vi "PPS_TRAJECTORY_EXECUTE_ABS.vi"(8 "Init":bool, 11 "End Pose ENG":T6={"TRANSLATION"={"X"=0.0, "Y"=0.0}, "ROTATION"={"VALUE"=0.0, "COS"=1.0, "SIN"=0.0}} {"ROTATION"."SIN" format="%13.4f"; "ROTATION"."COS" format="%13.4f"; "ROTATION"."VALUE" format="%13.4f"; "TRANSLATION"."Y" format="%14.3f"; "TRANSLATION"."X" format="%14.3f"}) -> (0 "AtReference":bool, 3 "Chassis Velocity Target SI":T7 {"vOmega" format="%10.3f"; "vY" format="%10.3f"; "vX" format="%10.3f"})   [LabVIEW 2019]
uses:
  <vilib>/Rock Robotics/WPI/ThirdParty/JAS_Junk/TrajLib/TypeDef/CHASSIS_SPEEDS.ctl
  <vilib>/Rock Robotics/WPI/ThirdParty/JAS_Junk/TrajLib/TypeDef/POSE2D.ctl
  <vilib>/Rock Robotics/WPI/ThirdParty/JAS_Junk/TrajLib/TypeDef/TRANSLATION2D.ctl
  <vilib>/Rock Robotics/WPI/ThirdParty/JAS_Junk/TrajLib/TypeDef/ROTATION2D.ctl
  <vilib>/Rock Robotics/WPI/ThirdParty/MJansen/PathPlanner/TypeDef/PathPlannerTrajectory.ctl
  <vilib>/Rock Robotics/WPI/ThirdParty/MJansen/PathPlanner/TypeDef/PathPlannerTrajectoryState.ctl
  <vilib>/Rock Robotics/WPI/ThirdParty/MJansen/PathPlanner/TypeDef/PathPlannerPathConstraints.ctl
  <vilib>/Rock Robotics/WPI/ThirdParty/JAS_Junk/TrajLib/VI/Util_GetTime_U32.vi
  <vilib>/Rock Robotics/WPI/ThirdParty/JAS_Junk/TrajLib/ProfiledPIDController_NewPeriod.vi
  <vilib>/Rock Robotics/WPI/ThirdParty/JAS_Junk/TrajLib/ProfiledPIDController_SetIntegratorRange.vi
  <vilib>/Rock Robotics/WPI/ThirdParty/JAS_Junk/TrajLib/ProfiledPIDController_DisableContInput.vi
  <vilib>/Rock Robotics/WPI/ThirdParty/JAS_Junk/TrajLib/ProfiledPIDController_EnableContInput.vi
  <vilib>/Rock Robotics/WPI/ThirdParty/JAS_Junk/TrajLib/TrapProfConstraint_New.vi
  <vilib>/Rock Robotics/WPI/ThirdParty/JAS_Junk/TrajLib/Pose2d_New.vi
  <vilib>/Rock Robotics/WPI/ThirdParty/JAS_Junk/TrajLib/Conv_Deg_Radians.vi
  <vilib>/Rock Robotics/WPI/ThirdParty/JAS_Junk/TrajLib/Rotation2d_UnaryMinus.vi
  <vilib>/Rock Robotics/WPI/ThirdParty/JAS_Junk/TrajLib/Rotation2d_RotateBy.vi
  <vilib>/Rock Robotics/WPI/ThirdParty/JAS_Junk/TrajLib/Rotation2d_GetRadians.vi
  <vilib>/Rock Robotics/WPI/ThirdParty/JAS_Junk/TrajLib/TrapProfState_New.vi
  <vilib>/Rock Robotics/WPI/ThirdParty/JAS_Junk/TrajLib/PIDController_NewPeriod.vi
  <vilib>/Rock Robotics/SystemInterfaces/NetworkCommunication/NetComm_UsageReport_report.vi
  <vilib>/Rock Robotics/WPI/ThirdParty/JAS_Junk/TrajLib/PIDController_SetIntegratorRange.vi
  <vilib>/Rock Robotics/WPI/ThirdParty/JAS_Junk/TrajLib/PIDController_DisableContinousInput.vi
  <vilib>/Rock Robotics/WPI/ThirdParty/JAS_Junk/TrajLib/PIDController_EnableContinousInput.vi
  <vilib>/Rock Robotics/WPI/ThirdParty/JAS_Junk/TrajLib/Rotation2d_CreateAngle.vi
  <vilib>/Rock Robotics/WPI/ThirdParty/JAS_Junk/TrajLib/Translation2d_Create.vi
  <vilib>/Rock Robotics/WPI/ThirdParty/JAS_Junk/TrajLib/Rotation2d_CreateXY.vi
  <vilib>/Rock Robotics/WPI/ThirdParty/JAS_Junk/TrajLib/Util_CalcDist.vi
  <vilib>/Rock Robotics/WPI/ThirdParty/JAS_Junk/TrajLib/VI/Util_GetTime_U64.vi
  PPS_TRAJECTORY_GLOBALS.vi
  Swerve_Drive_System/PPS_DRIVE_GLOBALS.vi
  <vilib>/Rock Robotics/WPI/ThirdParty/JAS_Junk/TrajLib/Globals/Util_LibraryGlobals.vi
  <vilib>/Rock Robotics/WPI/ThirdParty/JAS_Junk/TrajLib/Trajectory_Library.lvlib
  <vilib>/Rock Robotics/WPI/ThirdParty/MJansen/PathPlanner/PathPlanner24.lvlib
panel:
  out "PathPlannerTrajectory":T1 {"States"."TargetHolonomicRotation"."SIN" format="%13.4f"; "States"."TargetHolonomicRotation"."COS" format="%13.4f"; "States"."TargetHolonomicRotation"."VALUE" format="%13.4f"; "States"."Heading"."SIN" format="%13.4f"; "States"."Heading"."COS" format="%13.4f"; "States"."Heading"."VALUE" format="%13.4f"; "States"."PositionMeters"."Y" format="%14.3f"; "States"."PositionMeters"."X" format="%14.3f"}
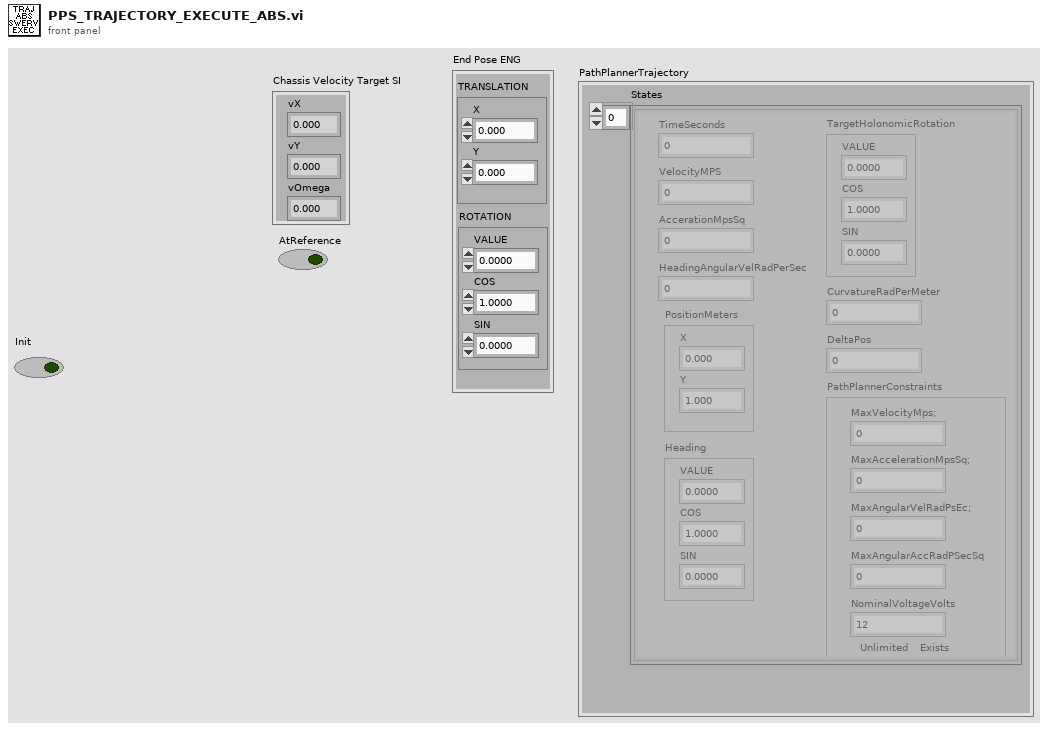
[diagram p1: front panel]
types:
  T1 = typedef "PathPlanner24.lvlib/PathPlannerTrajectory.ctl" = cluster{"States":T2[]}
  T2 = typedef "PathPlanner24.lvlib/PathPlannerTrajectoryState.ctl" = cluster{"TimeSeconds":dbl, "VelocityMPS":dbl, "AccerationMpsSq":dbl, "HeadingAngularVelRadPerSec":dbl, "PositionMeters":T3, "Heading":T4, "TargetHolonomicRotation":T4, "CurvatureRadPerMeter":dbl, "PathPlannerConstraints":T5, "DeltaPos":dbl}
  T3 = typedef "Trajectory_Library.lvlib/TRANSLATION2D.ctl" = cluster{"X":dbl, "Y":dbl}
  T4 = typedef "Trajectory_Library.lvlib/ROTATION2D.ctl" = cluster{"VALUE":dbl, "COS":dbl, "SIN":dbl}
  T5 = typedef "PathPlanner24.lvlib/PathPlannerPathConstraints.ctl" = cluster{"MaxVelocityMps;":dbl, "MaxAccelerationMpsSq;":dbl, "MaxAngularVelRadPsEc;":dbl, "MaxAngularAccRadPSecSq":dbl, "Exists":bool, "Unlimited":bool, "NominalVoltageVolts":dbl}
  T6 = typedef "Trajectory_Library.lvlib/POSE2D.ctl" = cluster{"TRANSLATION":T3, "ROTATION":T4}
  T7 = typedef "Trajectory_Library.lvlib/CHASSIS_SPEEDS.ctl" = cluster{"vX":dbl, "vY":dbl, "vOmega":dbl}
  T8 = typedef "Trajectory_Library.lvlib/SWERVE_DRIVE_KINEMATICS.ctl" = cluster{"NumModules":i32, "InverseKinematics":T9, "ForwardKinematics":T9, "Modules":T3[], "PrevCoR":T3, "SavedModuleStates":T10[]}
  T9 = typedef "NI_Matrix.lvlib/RealMatrix.ctl" = dbl[][]
  T10 = typedef "Trajectory_Library.lvlib/SWERVE_DRIVE_MODULE_STATE.ctl" = cluster{"Speed":dbl, "Angle":T4}
  T11 = typedef "Trajectory_Library.lvlib/PID_TUNING.ctl" = cluster{"Kp":dbl, "Ki":dbl, "Kd":dbl, "MaximumIntegral":dbl, "MinimumIntegral":dbl, "IntegralZone":dbl}
  T12 = typedef "Trajectory_Library.lvlib/PROFILED_PID_CONTROLLER.ctl" = cluster{"Controller":T13, "Goal":T14, "Setpoint":T14, "Constraint":T15}
  T13 = typedef "Trajectory_Library.lvlib/PID_CONTROLLER.ctl" = cluster{"Kp":dbl, "Ki":dbl, "Kd":dbl, "Period":dbl, "Max_Integral":dbl, "Min_Integral":dbl, "Max_Input":dbl, "Min_Input":dbl, "Continuous":bool, "PositionError":dbl, "VelocityError":dbl, "PrevError":dbl, "Total_Integral":dbl, "PositionTolerance":dbl, "VelocityTolerance":dbl, "SetPoint":dbl, "Kf":dbl, "Prev_Deriv":dbl, "Prev_Deriv 2":dbl, "DerivativeFilter":bool, "Min_Output":dbl, "Max_Output":dbl, "Prev_F_P":dbl, "Prev_F_P_2":dbl, "AntiWindupActive":bool, "Measurement":dbl, "IntegralZone":dbl}
  T14 = typedef "Trajectory_Library.lvlib/TRAPEZOID_PROFILE_STATE.ctl" = cluster{"Position":dbl, "Velocity":dbl}
  T15 = typedef "Trajectory_Library.lvlib/TRAPEZOID_PROFILE_CONSTRAINT.ctl" = cluster{"MaxVelocity":dbl, "MaxAcceleration":dbl}
  T16 = typedef "PathPlanner24.lvlib/PathPlannerCtrlHolConfig.ctl" = cluster{"HOLONOMIC_CTRL_PACK_TUNING":T17, "Max Wheel Speed M/S":dbl, "Tolerance SI":T6, "Drive Base Radius M":dbl}
  T17 = typedef "Trajectory_Library.lvlib/HOLONOMIC_PACK_TUNING.ctl" = cluster{"X PID Tuning":T11, "Y PID Tuning":T11, "thetaProfiledPID_CTRL":T12}
  T18 = typedef "Trajectory_Library.lvlib/HOLONOMIC_DRV_CTRL.ctl" = cluster{"poseTolerance":T6, "poseError":T6, "Enabled":bool, "PID_xCtrl":T13, "PID_yCtrl":T13, "PROF_PID_thetaCtrl":T12, "RotationError":T4, "FirstRun":bool}
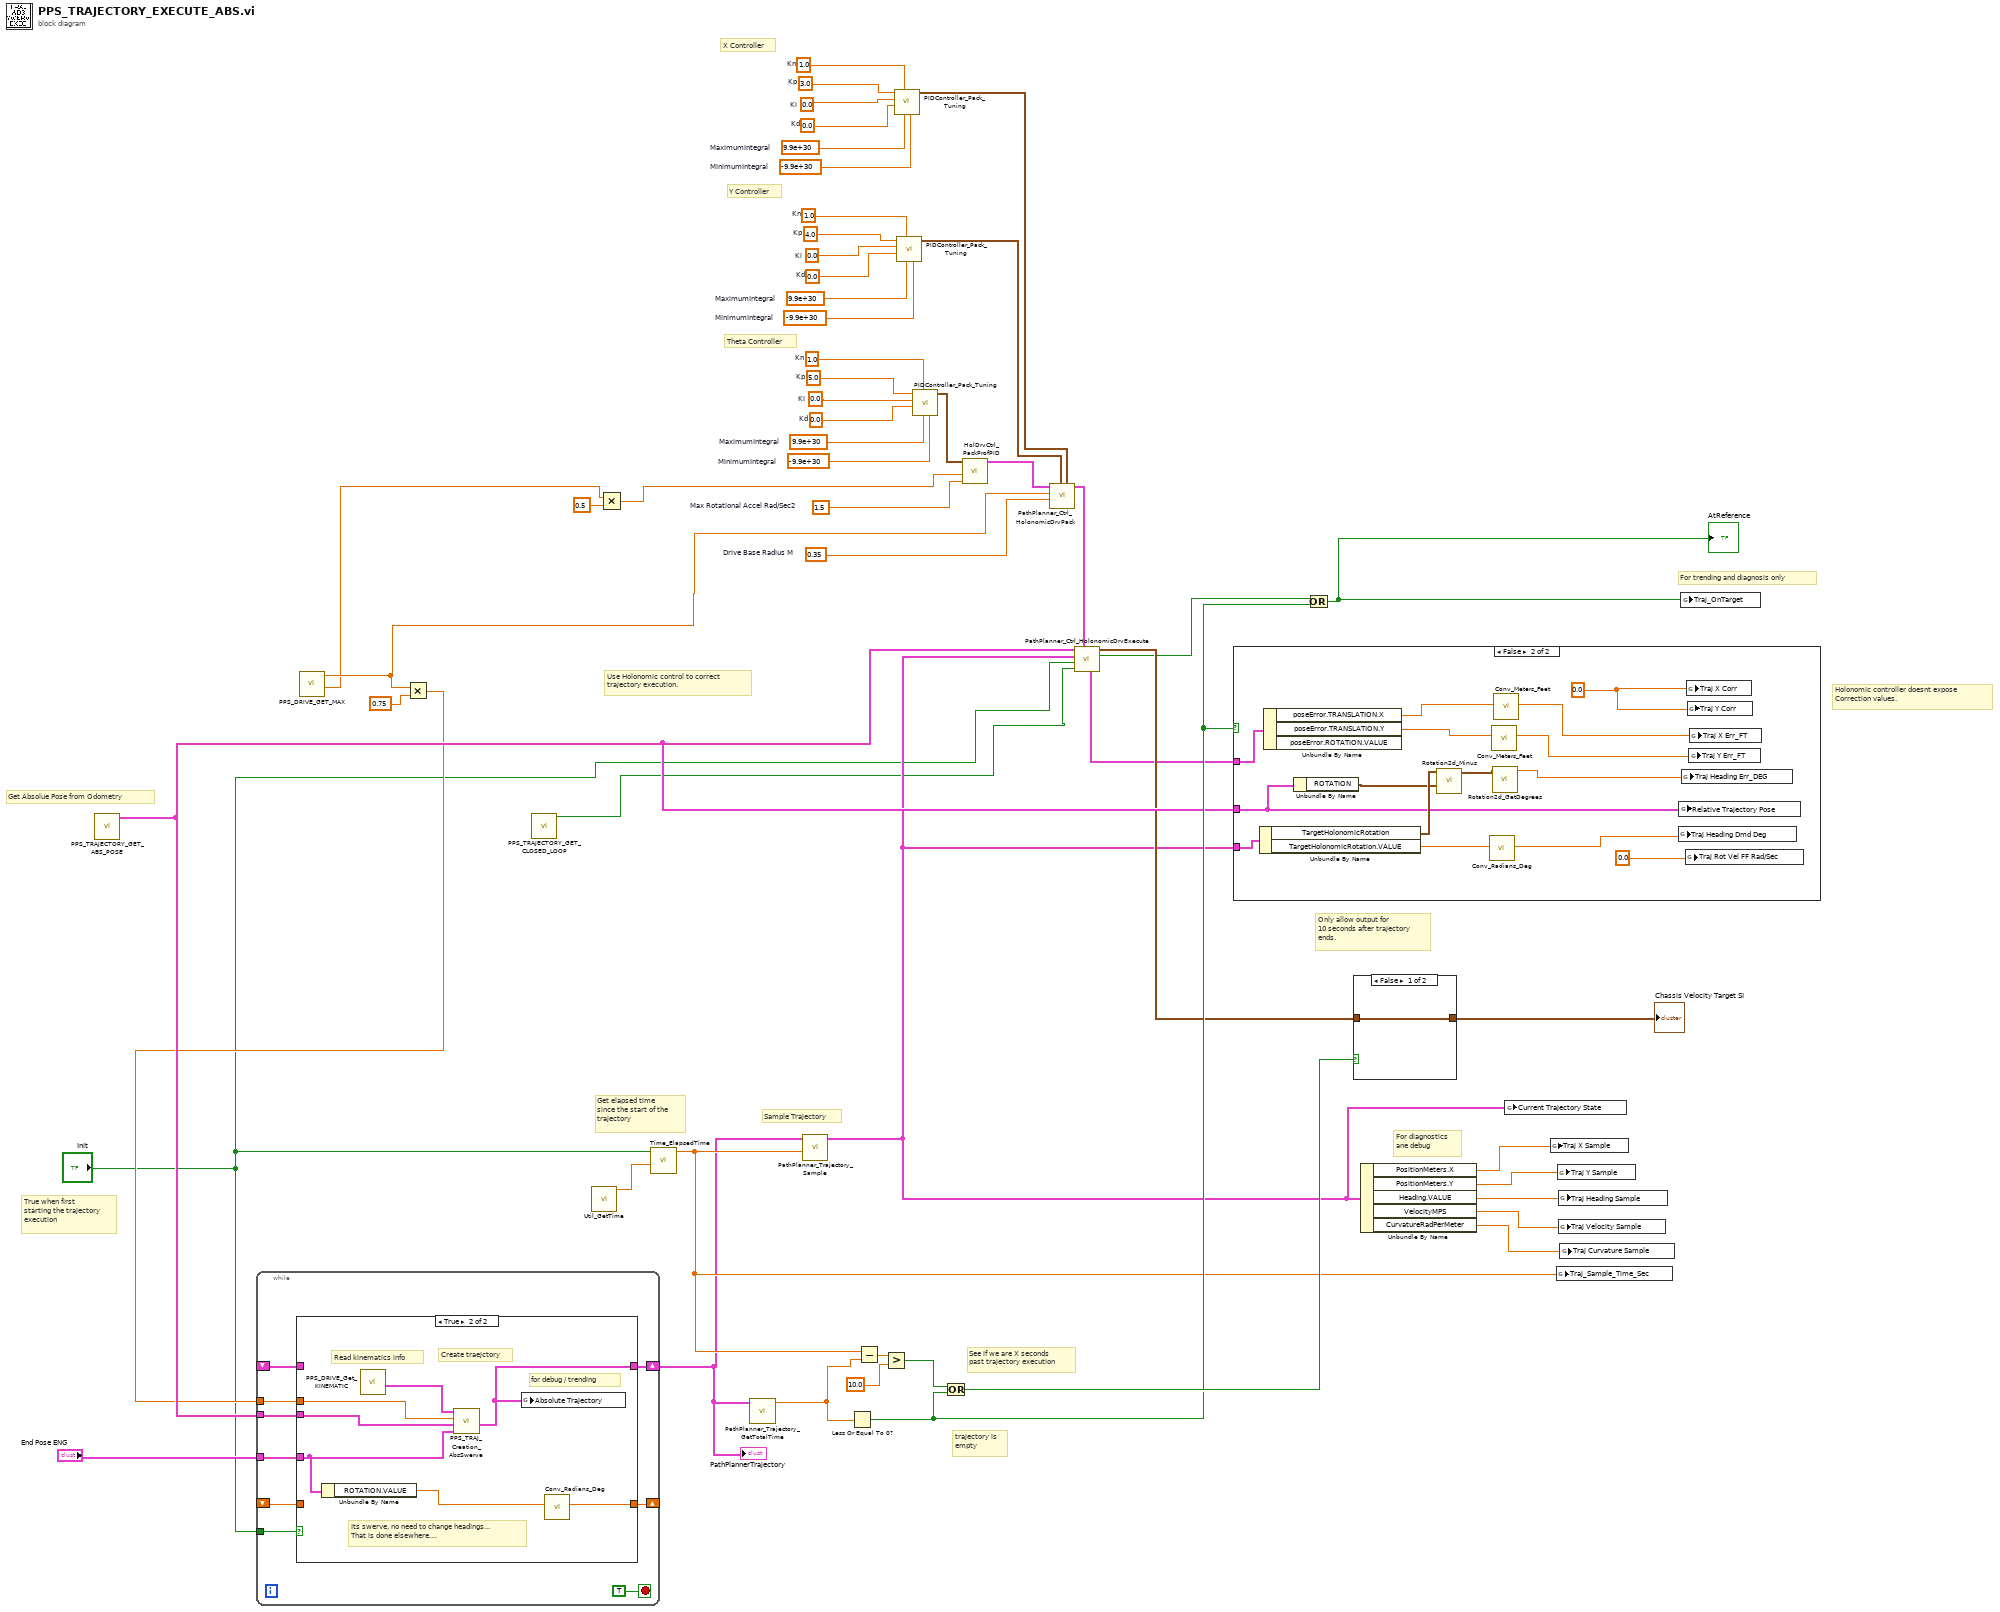
[diagram p0: block diagram]
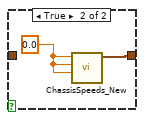
[diagram p4: hidden frame]
diagram:
  w32 = 0.35  # Drive Base Radius M
  w24 = 1.0  # Kn
  w21 = 5.0  # Kp
  w12 = 0.0  # Ki
  w11 = 0.0  # Kd
  w10 = 9.9e+30  # MaximumIntegral
  w9 = -9.9e+30  # MinimumIntegral
  w26 = 1.0  # Kn
  w23 = 3.0  # Kp
  w20 = 0.0  # Ki
  w19 = 0.0  # Kd
  w18 = 9.9e+30  # MaximumIntegral
  w17 = -9.9e+30  # MinimumIntegral
  w25 = 1.0  # Kn
  w22 = 4.0  # Kp
  w16 = 0.0  # Ki
  w15 = 0.0  # Kd
  w14 = 9.9e+30  # MaximumIntegral
  w13 = -9.9e+30  # MinimumIntegral
  w27 = 1.5  # Max Rotational Accel Rad/Sec2
  # "Theta Controller"
  # "Y Controller"
  # "X Controller"
  # "trajectory is \nempty"
  # "True when first\nstarting the trajectory\nexecution"
  # "Get elapsed time\nsince the start of the\ntrajectory"
  # "Holonomic controller doesnt expose\nCorrection values."
  # "Use Holonomic control to correct\ntrajectory execution."
  # "For trending and diagnosis only"
  # "For diagnostics\nane debug"
  # "Get Absolue Pose from Odometry"
  # "Sample Trajectory"
  # "See if we are X seconds \npast trajectory execution"
  # "Only allow output for\n10 seconds after trajectory\nends."
  n1 = call "PPS_TRAJECTORY_GET_ABS_POSE.vi"() -> ("Absolute Odometry Pose"=w40:T6)  [unwired: 11 in]
  n2 = call "PPS_DRIVE_GET_MAX.vi"() -> ("Max Rotational Vel (Rad/Sec)"=w5:dbl, "Max Wheel Vel (Meter/Sec)"=w7:dbl)  [unwired: 10 in]
  n3 = Multiply(x=w7, y=0.75) -> (x*y=w34:dbl)
  n4 = while {
    tunnel: "Init" -> [w63]
    tunnel: w40 -> [w62]
    shift-right: [w61] -> w37
    shift-left: _ -> [w60]
    shift-right: [w59] -> _
    shift-left: _ -> [w58]
    tunnel: "End Pose ENG" -> [w57]
    tunnel: w34 -> [w56]
    stop <- TRUE stop-if-true
    n5 = case shown="True" w63 {
      tunnel: w62 -> [_ w68]
      tunnel: [w66 w70] -> w61
      tunnel: w60 -> [w66 _]
      tunnel: [w65 w72] -> w59
      tunnel: w58 -> [w65 _]
      tunnel: w57 -> [_ w73]
      tunnel: w56 -> [_ w67]
      frame False {
      }
      frame True {
        # "for debug / trending"
        # "Read kinematics info"
        # "Its swerve, no need to change headings...\nThat is done elsewhere...."
        # "Create traejctory"
        n6 = Unbundle By Name(w73) -> ("ROTATION.VALUE"=w71:dbl)
        n7 = call "PPS_DRIVE_Get_KINEMATIC.vi"() -> ("out SWERVE_DRIVE_KINEMATICS"=w69:T8)  [unwired: 11 in]
        n8 = call "PPS_TRAJ_Creation_AbsSwerve.vi"("End Pose  ENG"=w73, "Current Pose SI"=w68, "Max Velocity M/S"=w67, "SWERVE_DRIVE_KINEMATICS"=w69) -> ("PathPlannerTrajectory"=w70:T1)  [unwired: 5 in, 2 out]
        n9 = global write "PPS_TRAJECTORY_GLOBALS.vi" "Absolute Trajectory"(w70) -> ()
        n10 = call <vilib>:"Conv_Radians_Deg.vi"("Radians"=w71) -> ("Degrees"=w72:dbl)  [unwired: 10 in]
      }
    }
  }
  "PathPlannerTrajectory" <- w37
  n11 = call "PPS_TRAJECTORY_GET_CLOSED_LOOP.vi"() -> ("AUTO_CLOSED_LOOP"=w1:bool)  [unwired: 11 in]
  n12 = call <vilib>:"Util_GetTime.vi"() -> ("FPGA_Time_Seconds"=w52:dbl)  [unwired: 9 in, 2 out]
  n13 = Multiply(x=w5, y=0.5) -> (x*y=w4:dbl)
  n14 = call <vilib>:"Time_ElapsedTime.vi"("PassthroughTime_SEC"=w52, "Reset"="Init") -> ("Elapsed Time Sec"=w41:dbl)  [unwired: 9 in]
  n15 = call <vilib>:"PathPlanner_Trajectory_GetTotalTime.vi"("PathPlannerTrajectory"=w37) -> ("TotalTimeSeconds"=w36:dbl)  [unwired: 10 in]
  n16 = call <vilib>:"PathPlanner_Trajectory_Sample.vi"("Time"=w41, "PathPlannerTrajectory"=w37) -> ("PathPlannerState"=w35:T2)  [unwired: 9 in]
  n17 = Less Or Equal To 0?(x=w36) -> (x <= 0?=w42:bool)
  n18 = Subtract(x=w41, y=w36) -> (x-y=w55:dbl)
  n19 = Greater?(x=w55, y=10.0) -> (0:w45:bool)
  n20 = call <vilib>:"PIDController_Pack_Tuning.vi"("MinimumIntegral"=w17, "MaximumIntegral"=w18, "Kn"=w26, "Kd"=w19, "Ki"=w20, "Kp"=w23) -> ("PID Tuning"=w29:T11)  [unwired: 5 in]
  n21 = call <vilib>:"PIDController_Pack_Tuning.vi"("MinimumIntegral"=w13, "MaximumIntegral"=w14, "Kn"=w25, "Kd"=w15, "Ki"=w16, "Kp"=w22) -> ("PID Tuning"=w30:T11)  [unwired: 5 in]
  n22 = call <vilib>:"PIDController_Pack_Tuning.vi"("MinimumIntegral"=w9, "MaximumIntegral"=w10, "Kn"=w24, "Kd"=w11, "Ki"=w12, "Kp"=w21) -> ("PID Tuning"=w28:T11)  [unwired: 5 in]
  n23 = Or(x=w45, y=w42) -> (x .or. y?=w44:bool)
  n24 = call <vilib>:"HolDrvCtrl_PackProfPID.vi"("Max Accel"=w27, "Max Speed"=w4, "Theta PID Tuning"=w28) -> ("Theta PID CONTROLLER"=w31:T12)  [unwired: 8 in]
  n25 = call <vilib>:"PathPlanner_Ctrl_HolonomicDrvPack.vi"("X PID Tuning"=w29, "Y PID Tuning"=w30, "Drive Base Radius M"=w32, "Max Wheel Speed M/S"=w7, "thetaProfiledPID_CTRL"=w31) -> ("PathPlanner_Ctrl_HolDrvConfig"=w8:T16)  [unwired: 6 in]
  n26 = call <vilib>:"PathPlanner_Ctrl_HolonomicDrvExecute.vi"("PathPlanner_Ctrl_HolDrvConfig"=w8, "Enabled"=w1, "Reset"="Init", "PathPlannerState"=w35, "Current Pose SI"=w40) -> ("At Reference"=w38:bool, "calcChassisSpeed"=w39:T7, "outHOLONOMIC_DRV_CTRL"=w6:T18)  [unwired: 3 in, 1 out]
  n27 = case shown="False" w42 {
    tunnel: w40 -> [_ w77]
    tunnel: w6 -> [_ w84]
    tunnel: w35 -> [_ w81]
    frame True {
    }
    frame False {
      w88 = 0.0 ("Y Corr")
      n28 = Unbundle By Name(w81) -> ("TargetHolonomicRotation"=w78:T4, "TargetHolonomicRotation.VALUE"=w80:dbl)
      n29 = Unbundle By Name(w84) -> ("poseError.TRANSLATION.X"=w83:dbl, "poseError.TRANSLATION.Y"=w82:dbl)  [unwired: 1 out]
      n30 = Unbundle By Name(w77) -> ("ROTATION"=w76:T4)
      n31 = call <vilib>:"Rotation2d_Minus.vi"("other ROTATION"=w76, "in ROTATION"=w78) -> ("out ROTATION"=w75:T4)  [unwired: 9 in]
      n32 = call <vilib>:"Conv_Radians_Deg.vi"("Radians"=w80) -> ("Degrees"=w79:dbl)  [unwired: 10 in]
      n33 = call <vilib>:"Conv_Meters_Feet.vi"("Meters"=w82) -> ("Feet"=w87:dbl)  [unwired: 10 in]
      n34 = call <vilib>:"Rotation2d_GetDegrees.vi"("in ROTATION"=w75) -> ("AngleDegrees"=w74:dbl)  [unwired: 10 in]
      n35 = call <vilib>:"Conv_Meters_Feet.vi"("Meters"=w83) -> ("Feet"=w86:dbl)  [unwired: 10 in]
      n36 = global write "PPS_TRAJECTORY_GLOBALS.vi" "Traj Heading Dmd Deg"(w79) -> ()
      n37 = global write "PPS_TRAJECTORY_GLOBALS.vi" "Relative Trajectory Pose"(w77) -> ()
      n38 = global write "PPS_TRAJECTORY_GLOBALS.vi" "Traj Heading Err_DEG"(w74) -> ()
      n39 = global write "PPS_TRAJECTORY_GLOBALS.vi" "Traj Rot Vel FF Rad/Sec"(0.0 ("Traj Heading Dmd Deg")) -> ()
      n40 = global write "PPS_TRAJECTORY_GLOBALS.vi" "Traj X Corr"(w88) -> ()
      n41 = global write "PPS_TRAJECTORY_GLOBALS.vi" "Traj Y Corr"(w88) -> ()
      n42 = global write "PPS_TRAJECTORY_GLOBALS.vi" "Traj Y Err_FT"(w87) -> ()
      n43 = global write "PPS_TRAJECTORY_GLOBALS.vi" "Traj X Err_FT"(w86) -> ()
    }
  }
  n44 = Or(x=w38, y=w42) -> (x .or. y?=w43:bool)
  "AtReference" <- w43
  n45 = case shown="False" w44 {
    tunnel: w39 -> [w89 _]
    tunnel: [w89 w90] -> w53
    frame False {
    }
    frame True {
      w91 = 0.0 ("vX")
      n46 = call <vilib>:"ChassisSpeeds_New.vi"("vAngular"=w91, "vY"=w91, "vX"=w91) -> ("CHASSIS"=w90:T7)  [unwired: 8 in]
    }
  }
  "Chassis Velocity Target SI" <- w53
  n47 = Unbundle By Name(w35) -> ("PositionMeters.X"=w51:dbl, "PositionMeters.Y"=w50:dbl, "Heading.VALUE"=w49:dbl, "VelocityMPS"=w48:dbl, "CurvatureRadPerMeter"=w47:dbl)
  n48 = global write "PPS_TRAJECTORY_GLOBALS.vi" "Current Trajectory State"(w35) -> ()
  n49 = global write "PPS_TRAJECTORY_GLOBALS.vi" "Traj X Sample"(w51) -> ()
  n50 = global write "PPS_TRAJECTORY_GLOBALS.vi" "Traj_Sample_Time_Sec"(w41) -> ()
  n51 = global write "PPS_TRAJECTORY_GLOBALS.vi" "Traj Y Sample"(w50) -> ()
  n52 = global write "PPS_TRAJECTORY_GLOBALS.vi" "Traj Heading Sample"(w49) -> ()
  n53 = global write "PPS_TRAJECTORY_GLOBALS.vi" "Traj Velocity Sample"(w48) -> ()
  n54 = global write "PPS_TRAJECTORY_GLOBALS.vi" "Traj Curvature Sample"(w47) -> ()
  n55 = global write "PPS_TRAJECTORY_GLOBALS.vi" "Traj_OnTarget"(w43) -> ()
